vi "moveFilterWheel.vi"(6 "Delay between send and receive [ms]":i32=100, 8 "error in (no error)":errorcluster, 9 "position":i32, 10 "locationId":T1, 11 "Monochromator in":refnum<class "Monochromator.lvclass">) -> (0 "error out":errorcluster, 1 "ID":i32, 2 "results-JSON string":string, 3 "Monochromator out":refnum<class "Monochromator.lvclass">)   [LabVIEW 2023, in "Monochromator.lvclass"]
uses:
  Monochromator.lvclass
  CCD/FilterWheelLocationEnum.ctl
  29a0d797-fd6c-43e0-b242-80b21aa51c30.vi
  7fe8abea-6ecd-46de-aa11-ce8637911b6a.vi
  35d46a5a-fd7c-4445-96f4-e877dae8f93b.vi
  <vilib>/JDP Science/JSONtext/Variant to JSON Text.vi
  <vilib>/JDP Science/JSONtext/Set Item.vi
  <vilib>/JDP Science/JSONtext/LVClass Serializer/JSONtext LVClass Serializer.lvclass
  Monochromator.lvclass/Monochromator.ctl
  GenericDevice/GenericDevice.lvclass
  <vilib>/IlluminatedG/lv-web-crypto/lv-json/JSON/JSON.lvlib
panel:
  # "Connector Pane"
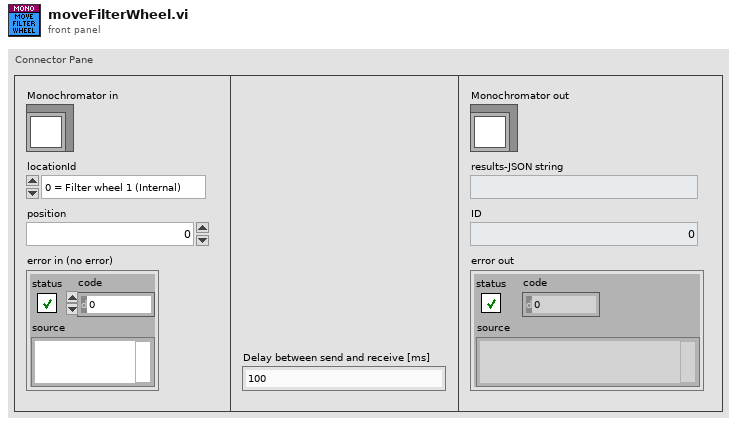
[diagram p1: front panel]
types:
  T1 = typedef "Monochromator.lvclass/FilterWheelLocationEnum.ctl" = enum16{"0 = Filter wheel 1 (Internal)", "1 = Filter wheel 2 (External)"}
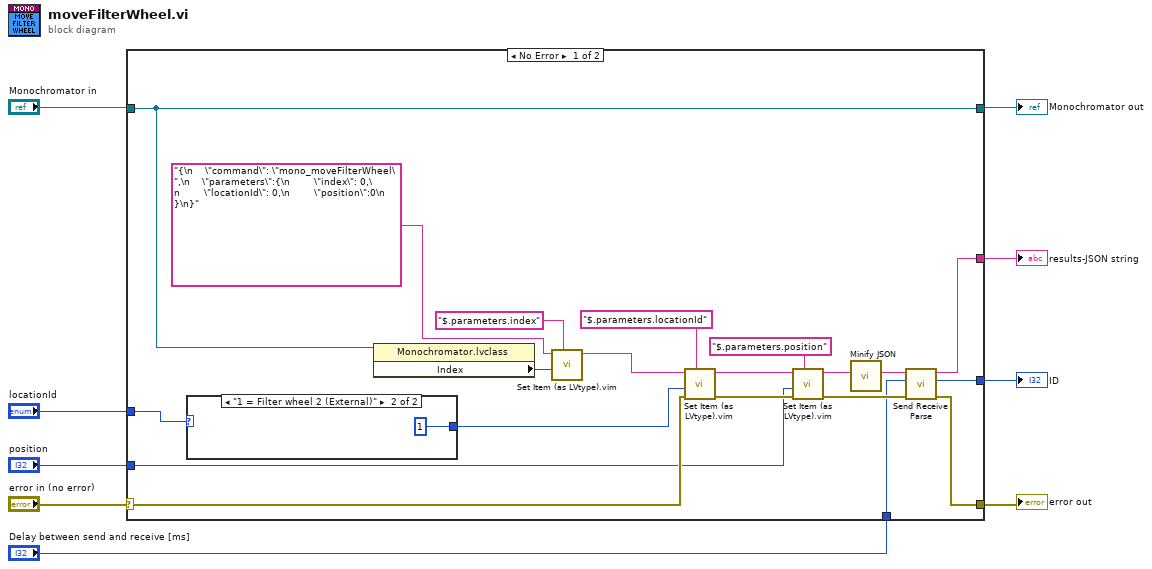
[diagram p0: block diagram]
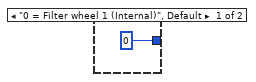
[diagram p2: hidden frame]
diagram:
  n1 = case shown="No Error" "error in (no error)" {
    selector: "error in (no error)" -> [w28 w33]
    tunnel: [w25 w33] -> w6
    tunnel: [w14 w32] -> w8
    tunnel: "Monochromator in" -> [w14 w32]
    tunnel: [w27 _] -> w4
    tunnel: [w26 _] -> w5
    tunnel: "position" -> [w18 _]
    tunnel: "locationId" -> [w16 _]
    tunnel: "Delay between send and receive [ms]" -> [w17 _]
    frame No Error {
      n2 = case shown="\"1 = Filter wheel 2 (External)\"" w16 {
        tunnel: [0 1] -> w15
        frame "0 = Filter wheel 1 (Internal)", Default {
        }
        frame "1 = Filter wheel 2 (External)" {
        }
      }
      n3 = property class="Monochromator.lvclass"(reference=w14) -> ("Index"=w13:i32)  [unwired: 1 in, 2 out]
      n4 = call "Set Item (as LVtype).vim"("$Path or Item Name"="$.parameters.index", "Anything"=w13, "JSON"="{\n    \"command\": \"mono_moveFilterWheel\",\n    \"parameters\":{\n        \"index\": 0,\n        \"locationId\": 0,\n        \"position\":0\n    }\n}") -> ("<JSON>"=w11:string)  [unwired: 5 in, 2 out]
      n5 = call "Set Item (as LVtype).vim"("$Path or Item Name"="$.parameters.locationId", "error in (no error)"=w28, "Anything"=w15, "JSON"=w11) -> ("error out"=w22:errorcluster, "<JSON>"=w20:string)  [unwired: 4 in, 1 out]
      n6 = call "Set Item (as LVtype).vim"("$Path or Item Name"="$.parameters.position", "error in (no error)"=w22, "Anything"=w18, "JSON"=w20) -> ("error out"=w21:errorcluster, "<JSON>"=w19:string)  [unwired: 4 in, 1 out]
      n7 = call <vilib>:"Minify JSON.vi"("JSON String"=w19) -> ("Minified JSON"=w24:string)  [unwired: 10 in]
      n8 = call "Send Receive Parse.vi"("error in"=w21, "Delay between send and receive [ms]"=w17, "<JSON>"=w24) -> ("error out"=w25:errorcluster, "ID"=w26:i32, "results-JSON string"=w27:string)  [unwired: 6 in]
    }
    frame Error {
    }
  }
  "error out" <- w6
  "Monochromator out" <- w8
  "ID" <- w5
  "results-JSON string" <- w4
